vi "gl_RefPlotRefreshRate.vi"() -> ()   [LabVIEW 2020]
panel:
  in  "Ref Plot refresh rate":dbl
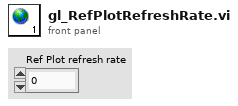
[diagram p1: front panel]
diagram:
